vi "Read files C CH1(Recorder).vi"(10 "Path":path, 11 "Number":dbl) -> (3 "Current":dbl format="%.4g")   [LabVIEW 2020, in "GPP.lvlib"]
uses:
  GPP.lvlib
panel:
  out "String":string
  out "String 2":string
  out "String 3":string
  out "Array":u8[](array[numeric])
  out "Numeric":u16
  out "C1":string
  out "V1 2":string
  out "LAST1":string
  out "SET":string
  out "ALL":string
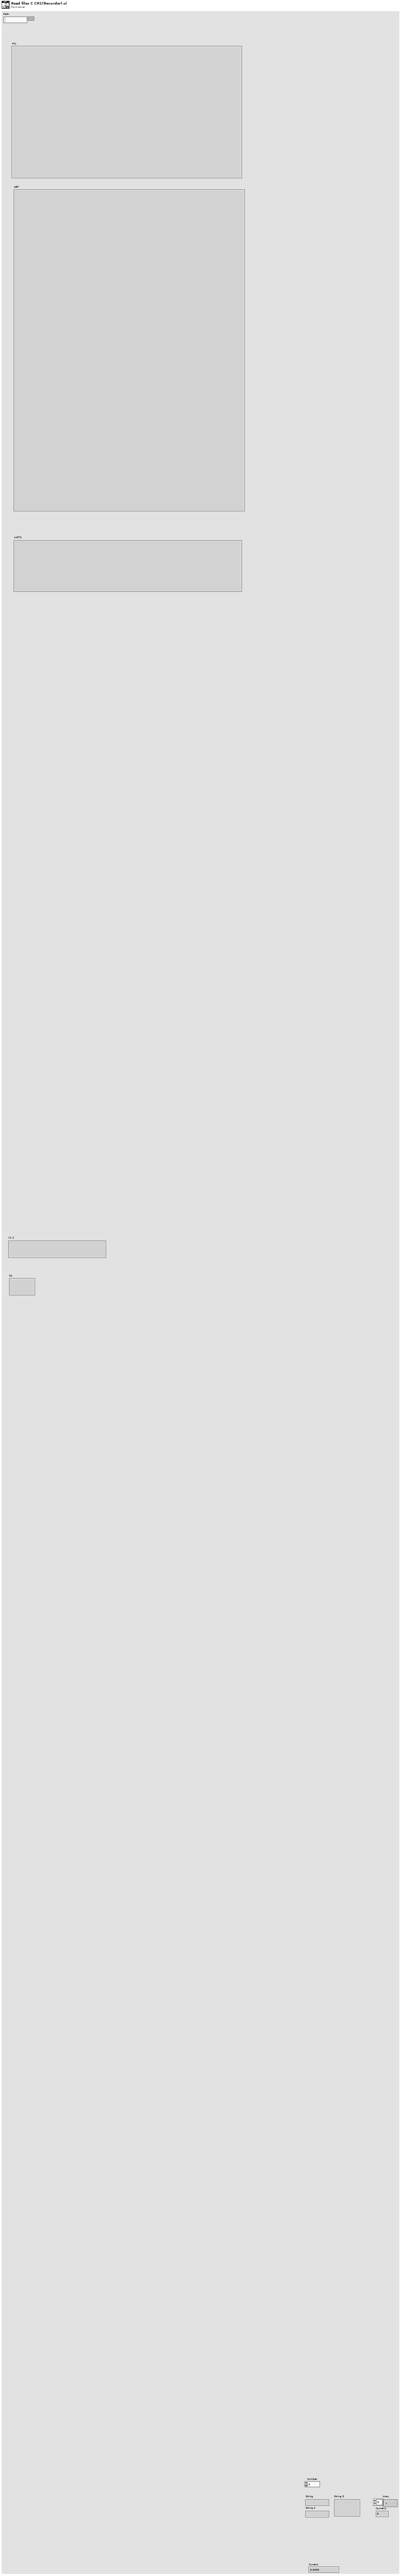
[diagram p1: front panel]
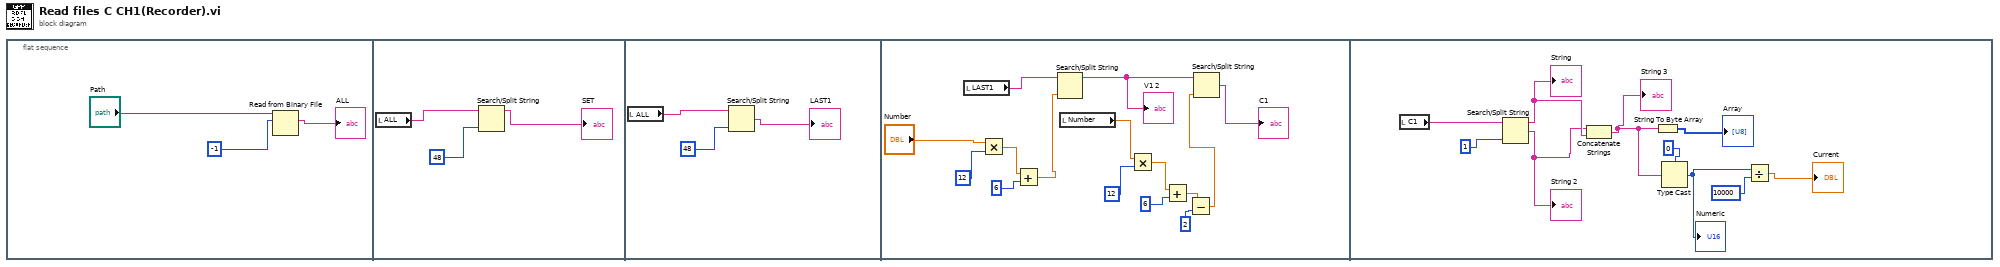
[diagram p0: block diagram]
diagram:
  n1 = flat-sequence {
    frame #0 {
      n2 = Read from Binary File(10:-1, 11:"Path") -> (2:→"ALL":string)  [unwired: 4 in, 3 out]
    }
    frame #1 {
      n3 = local read "ALL"() -> (w4:string)
      n4 = Search/Split String(string=w4, offset (0)=48) -> (substring before match=→"SET":string)  [unwired: 1 in, 2 out]
    }
    frame #2 {
      n5 = local read "ALL"() -> (w7:string)
      n6 = Search/Split String(string=w7, offset (0)=48) -> (match + rest of string=→"LAST1":string)  [unwired: 1 in, 2 out]
    }
    frame #3 {
      n7 = local read "LAST1"() -> (w21:string)
      n8 = Multiply(x="Number", y=12) -> (x*y=w20:dbl)
      n9 = Add(x=w20, y=6) -> (x+y=w10:dbl)
      n10 = Search/Split String(string=w21, offset (0)=w10) -> (substring before match=w14:string)  [unwired: 1 in, 2 out]
      "V1 2" <- w14
      n11 = local read "Number"() -> (w15:dbl)
      n12 = Multiply(x=w15, y=12) -> (x*y=w17:dbl)
      n13 = Add(x=w17, y=6) -> (x+y=w13:dbl)
      n14 = Subtract(x=w13, y=2) -> (x-y=w11:dbl)
      n15 = Search/Split String(string=w14, offset (0)=w11) -> (match + rest of string=→"C1":string)  [unwired: 1 in, 2 out]
    }
    frame #4 {
      n16 = local read "C1"() -> (w34:string)
      n17 = Search/Split String(string=w34, offset (0)=1) -> (substring before match=w32:string, match + rest of string=w31:string)  [unwired: 1 in, 1 out]
      "String" <- w32
      "String 2" <- w31
      n18 = Concatenate Strings(w31, w32) -> (w29:string)
      "String 3" <- w29
      n19 = String To Byte Array(string=w29) -> (unsigned byte array=→"Array":u8[])
      n20 = Type Cast(type=u16 0, x=w29) -> (*(type *) &x=w27:u16)
      "Numeric" <- w27
      n21 = Divide(x=w27, y=10000) -> (x/y=→"Current":dbl)
    }
  }
